vi "Select_data.vi"(7 "condition":string, 8 "error in (no error)":errorcluster caption="错误输入（无错误）", 9 "columns":string[](array[string]), 10 "table":string, 11 "access 输入":refnum<class "access.lvclass">) -> (0 "error out":errorcluster caption="错误输出", 2 "data":string[][](array[string]), 3 "access 输出":refnum<class "access.lvclass">)   [LabVIEW 2016, in "中水三立SQL数据传输.lvlib" / "access.lvclass"]
uses:
  access.lvclass
  <vilib>/addons/database/_DB Variant To Data/Database Variant To Data.xnode
  <vilib>/addons/database/NI_Database_API.lvlib
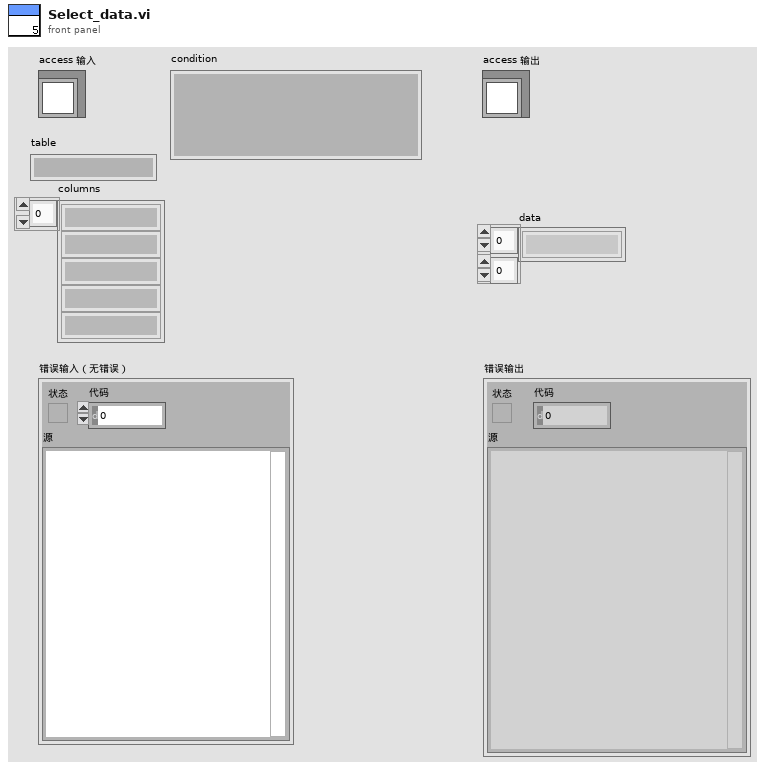
[diagram p1: front panel]
types:
  T1 = typedef "NI_Database_API.lvlib/Conn ObjectReference.ctl" = refnum<k1>
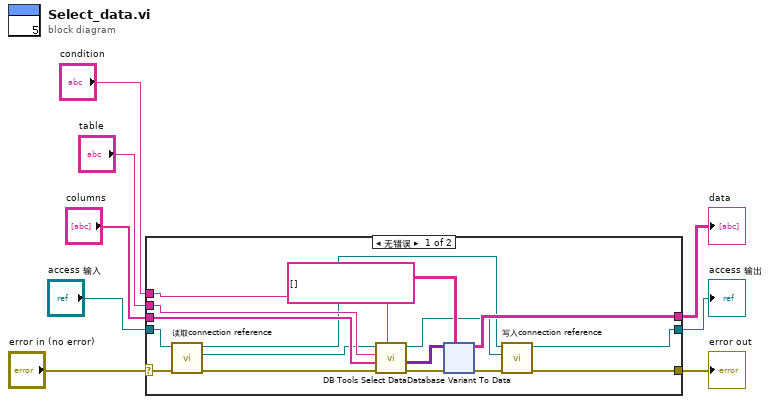
[diagram p0: block diagram]
diagram:
  n1 = case shown="无错误" "error in (no error)" {
    selector: "error in (no error)" -> [w15 w69]
    tunnel: "access 输入" -> [w17 w70]
    tunnel: "columns" -> [w23 _]
    tunnel: "table" -> [w22 _]
    tunnel: "condition" -> [w21 _]
    tunnel: [w18 _] -> w3
    tunnel: [w9 w69] -> w2
    tunnel: [w10 w70] -> w1
    frame No Error {
      n2 = call-dynamic "读取connection reference.vi"("error in (no error)"=w15, "database输入"=w17) -> ("error out"=w14:errorcluster, "reference"=w16:T1, "database输出"=w13:refnum<class "access.lvclass">)  [unwired: 7 in]
      n3 = call <vilib>:"DB Tools Select Data.vi"("condition"=w21, "error in (no error)"=w14, "columns"=w23, "table"=w22, "connection reference"=w16) -> ("error out"=w24:errorcluster, "data"=w20:variant[][], "connection reference out"=w12:T1)  [unwired: 1 in]
      n4 = xnode "Database Variant To Data"("database variant"=w20, "error in (no error)"=w24, "type"=string[][] []) -> ("data"=w18:string[][], "error out"=w11:errorcluster)
      n5 = call-dynamic "写入connection reference.vi"("error in (no error)"=w11, "reference"=w12, "database输入"=w13) -> ("error out"=w9:errorcluster, "database输出"=w10:refnum<class "access.lvclass">)  [unwired: 7 in]
    }
    frame Error {
    }
  }
  "error out" <- w2
  "access 输出" <- w1
  "data" <- w3
